vi "1TableHeaderFormatter.vi"(8 "error in (no error)":errorcluster, 10 "Data Name":string, 11 "HeaderPrefix":string) -> (0 "error out":errorcluster, 3 "HeaderOut":string)   [LabVIEW 2014, in "TableLogger_Actor.lvlib" / "TableLogger_Actor.lvclass"]
uses:
  TableLogger_Actor.lvclass
panel:
  # "Connector Pane"
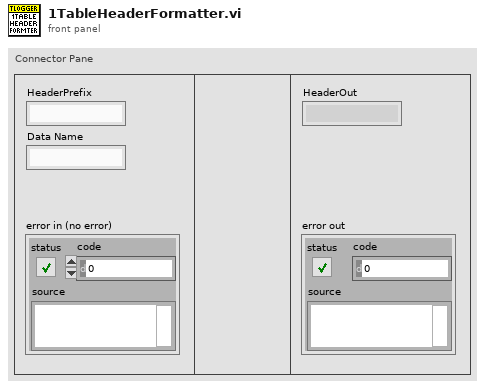
[diagram p1: front panel]
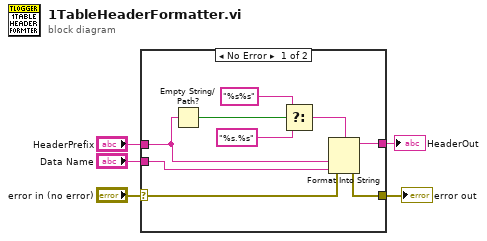
[diagram p0: block diagram]
diagram:
  n1 = case shown="No Error" "error in (no error)" {
    selector: "error in (no error)" -> [w14 w15]
    tunnel: [w13 w15] -> w4
    tunnel: [w12 _] -> w3
    tunnel: "Data Name" -> [w11 _]
    tunnel: "HeaderPrefix" -> [w7 _]
    frame No Error {
      n2 = Empty String/Path?(string/path=w7) -> (empty?=w10:bool)
      n3 = Select(t="%s%s" ("format string"), s=w10, f="%s.%s" ("format string")) -> (s? t:f=w6:string)
      n4 = Format Into String(format string=w6, error in=w14, w7, w11) -> (resulting string=w12:string, error out=w13:errorcluster)  [unwired: 1 in]
    }
    frame Error {
    }
  }
  "error out" <- w4
  "HeaderOut" <- w3
